vi "AlazarCreateStreamFile.vi"(2 "error in (no error)":errorcluster, 3 "File Path":string, 4 "Handle":u64) -> (0 "error out":errorcluster, 1 "Handle":u64)   [LabVIEW 2009]
doc: "Create a binary data file for this board, and enable saving AutoDMA data from this board to disk."
uses:
  ATSApi.dll
panel:
  out "Error Code":u32
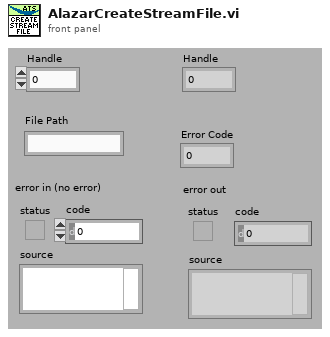
[diagram p1: front panel]
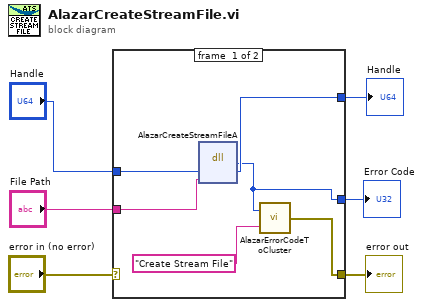
[diagram p0: block diagram]
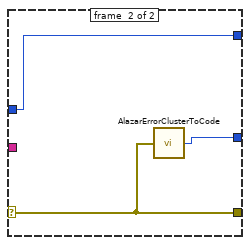
[diagram p2: hidden frame]
diagram:
  n1 = case shown="No Error" "error in (no error)" {
    selector: "error in (no error)" -> [_ w15]
    tunnel: [w10 w15] -> w5
    tunnel: "Handle" -> [w12 w14]
    tunnel: [w11 w14] -> w3
    tunnel: "File Path" -> [w9 _]
    tunnel: [w8 w13] -> w1
    frame #0 {
      n2 = dll-call lib="ATSApi.dll" fn="AlazarCreateStreamFileA"("handle"=w12, "filePath"=w9) -> ("return type"=w8:u32, "handle"=w11:u64)  [unwired: 4 in, 2 out]
      n3 = call "AlazarErrorCodeToCluster.vi"("Message"="Create Stream File", "Error Code"=w8) -> ("error out"=w10:errorcluster)
    }
    frame #1 {
      n4 = call "AlazarErrorClusterToCode.vi"("error in (no error)"=w15) -> ("Error Code"=w13:u32)
    }
  }
  "Handle" <- w3
  "error out" <- w5
  "Error Code" <- w1
